vi "Replace zero motor out if not stop.vi"(10 "Input":dbl, 11 "Stop?":bool) -> (3 "Output":dbl)   [LabVIEW 2017]
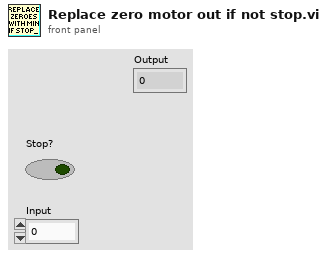
[diagram p1: front panel]
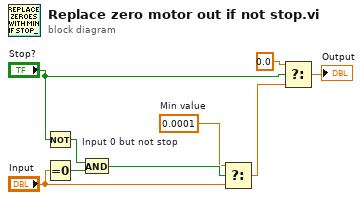
[diagram p0: block diagram]
diagram:
  w5 = 0.0001  # Min value
  n1 = Not(x="Stop?") -> (.not. x?=w7:bool)
  n2 = Equal To 0?(x="Input") -> (x = 0?=w8:bool)
  n3 = And "Input 0 but not stop"(x=w7, y=w8) -> (x .and. y?=w6:bool)
  n4 = Select(t=w5, s=w6, f="Input") -> (s? t:f=w3:dbl)
  n5 = Select(t=0.0, s="Stop?", f=w3) -> (s? t:f=→"Output":dbl)
